vi "CreatePrivateEvents.vi"(8 "error in (no error)":errorcluster, 11 "Logger":refnum<class "Logger.DSC.lvclass">) -> (0 "error out":errorcluster, 3 "Logger out":refnum<class "Logger.DSC.lvclass">)   [LabVIEW 2016, in "Logger.DSC.lvclass"]
doc: "---------------------------------------------------------------\nJKI State Machine Objects™\nhttp://jki.net/state-machine-objects/\nCopyright (C) 2005-2015, JKI <info@jki.net>\nALL RIGHTS RESERVEDJKI State Machine Objects (SMO) 1.0.0.4\nJKI - JKI\nCopyright (c) 2015, JKI"
uses:
  Logger.DSC.lvclass
  Typedefs/PrivateEvents--Logger.DSC.Set Address.ctl
  Typedefs/PrivateEvents--Logger.DSC.Write Variable.ctl
  Logger/Logger.lvclass
panel:
  # "For instructions on how to use the JKI State Machine Objects, examples and video tutorials, visit:\nhttp://jki.net/state-machine-objects/\n\nJKI State Machine Objects™\nhttp://jki.net/state-machine-objects/\nCopyright (C) 2005-2015, JKI <info@jki.net>\nALL RIGHTS RESERVED"
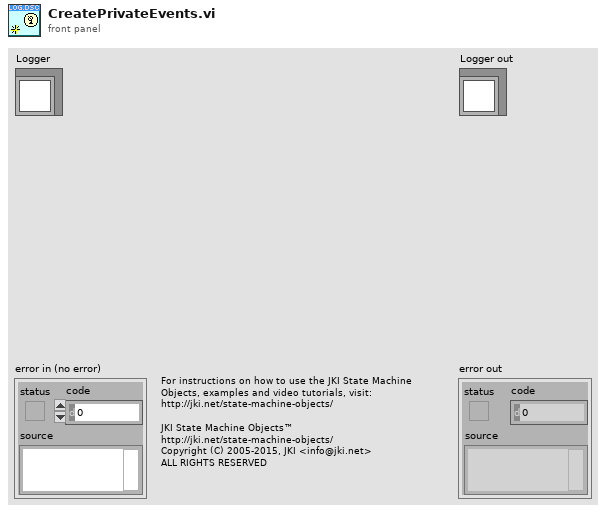
[diagram p1: front panel]
types:
  T1 = typedef "Logger.DSC.lvclass/PrivateEvents--Logger.DSC.Write Variable.ctl" = cluster{"Address":string, "Data":variant}
  T2 = typedef "Logger.DSC.lvclass/PrivateEvents--Logger.DSC.Set Address.ctl" = string
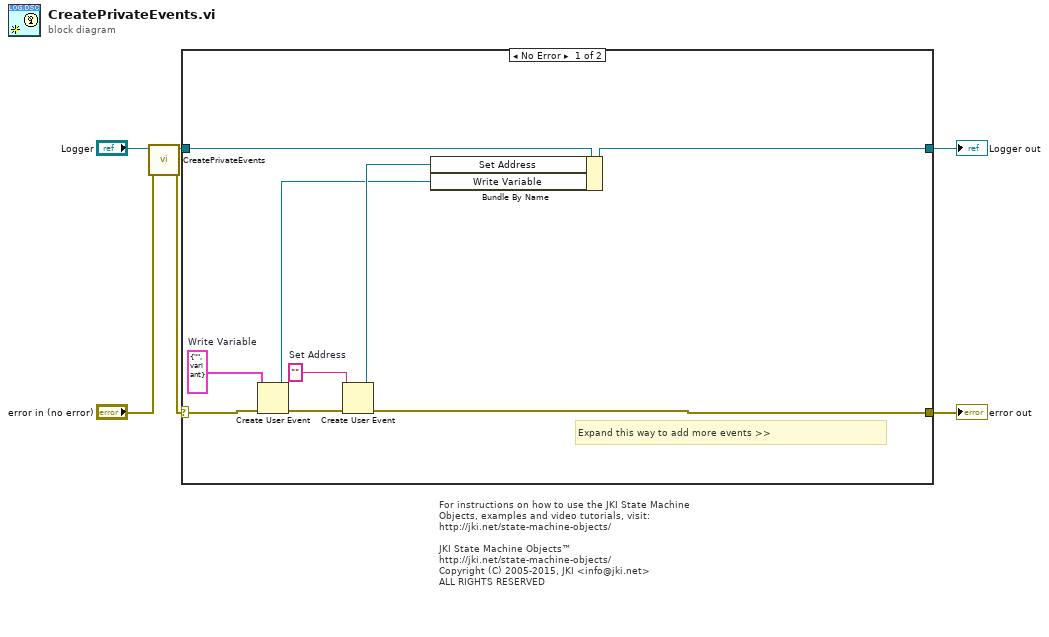
[diagram p0: block diagram]
diagram:
  # "For instructions on how to use the JKI State Machine Objects, examples and video tutorials, visit:\nhttp://jki.net/state-machine-objects/\n\nJKI State Machine Objects™\nhttp://jki.net/state-machine-objects/\nCopyright (C) 2005-2015, JKI <info@jki.net>\nALL RIGHTS RESERVED"
  n1 = call-parent "CreatePrivateEvents.vi"("error in (no error)"="error in (no error)", "SMO"="Logger") -> ("error out"=w1:errorcluster, "SMO out"=w3:refnum<class "Logger.DSC.lvclass">)  [unwired: 8 in]
  n2 = case shown="No Error" w1 {
    selector: w1 -> [w14 w17]
    tunnel: [w12 w17] -> w5
    tunnel: [w13 w16] -> w6
    tunnel: w3 -> [w15 w16]
    frame No Error {
      w8 = T1 {"Address"="", "Data"=variant(dbl 0.0)}  # Write Variable
      w11 = T2 ""  # Set Address
      # "Expand this way to add more events >>"
      n3 = Create User Event(user event datatype=w8, error in=w14) -> (user event=w7:refnum<user-event>, error out=w9:errorcluster)
      n4 = Create User Event(user event datatype=w11, error in=w9) -> (user event=w10:refnum<user-event>, error out=w12:errorcluster)
      n5 = Bundle By Name(cluster=w15, "Set Address"=w10, "Write Variable"=w7) -> (w13:refnum<class "Logger.DSC.lvclass">)
    }
    frame Error {
    }
  }
  "error out" <- w5
  "Logger out" <- w6
